vi "Protection_Valid_Calculation.vi"(8 "error in":errorcluster, 10 "Signal Settings":T1 {"Protection Configuration"."CRC Channels"."Data Type" items=["Signed", "Unsigned", "IEEE Float"]}, 11 "Signal Values In":dbl[](array[numeric])) -> (0 "error out":errorcluster, 3 "Signal Values Out":dbl[](array[numeric]))   [LabVIEW 2015, in "Protection and Counter Addon Engine.lvlib"]
uses:
  Protection and Counter Addon Engine.lvlib
  SubModules/Frame Protection Support/Source/Shared/Types/RT Exported Signal Settings.ctl
  SubModules/Frame Protection Support/Source/Shared/Types/Exported Counter Settings.ctl
  SubModules/Frame Protection Support/Source/Engine/Types/RT Protection Configuration.ctl
  SubModules/Frame Protection Support/Source/Shared/Types/Protection Type.ctl
  SubModules/Frame Protection Support/Source/Shared/Types/XNET Signal Configuration.ctl
  <vilib>/xnet/xnet.llb/XNET Convert (Signal to Frame Raw).vi
  SubModules/Frame Protection Support/Source/Shared/Protection and Counter Support Shared.lvlib
  SubModules/Frame Protection Support/Source/Engine/Protection and Counter Support Engine.lvlib
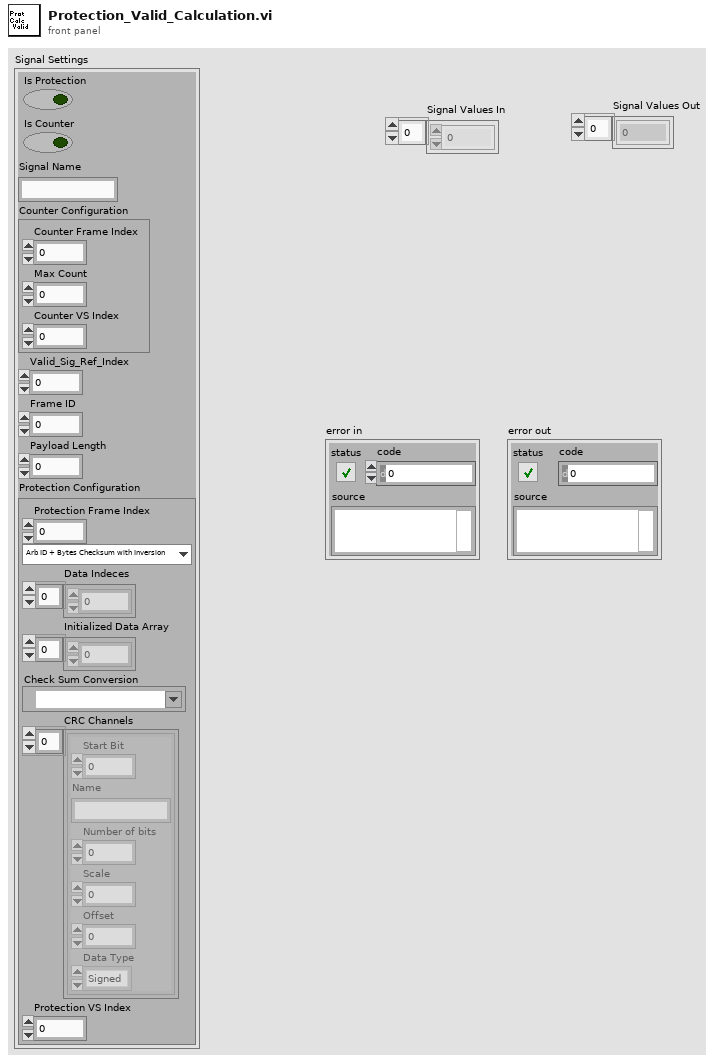
[diagram p1: front panel]
types:
  T1 = typedef "Protection and Counter Support Shared.lvlib/RT Exported Signal Settings.ctl" = cluster{"Is Protection":bool, "Is Counter":bool, "Signal Name":string, "Counter Configuration":T2, "Valid_Sig_Ref_Index":i32, "Frame ID":u32, "Payload Length":u32, "Protection Configuration":T3}
  T2 = typedef "Protection and Counter Support Shared.lvlib/Exported Counter Settings.ctl" = cluster{"Counter Frame Index":i32, "Max Count":dbl, "Counter VS Index":i32}
  T3 = typedef "Protection and Counter Support Engine.lvlib/RT Protection Configuration.ctl" = cluster{"Protection Frame Index":i32, "Protection Type":T4, "Data Indeces":i32[], "Initialized Data Array":dbl[], "Check Sum Conversion":refnum<k21>, "CRC Channels":T5[], "Protection VS Index":i32}
  T4 = typedef "Protection and Counter Support Shared.lvlib/Protection Type.ctl" = enum16{"Arb ID + Bytes Checksum with Inversion", "Arb ID + Bytes CRC with Inversion", "Reversed Raw Signal Checksum with Inversion"}
  T5 = typedef "Protection and Counter Support Shared.lvlib/XNET Signal Configuration.ctl" = cluster{"Start Bit":i32, "Name":string, "Number of bits":i32, "Scale":dbl, "Offset":dbl, "Data Type":u32}
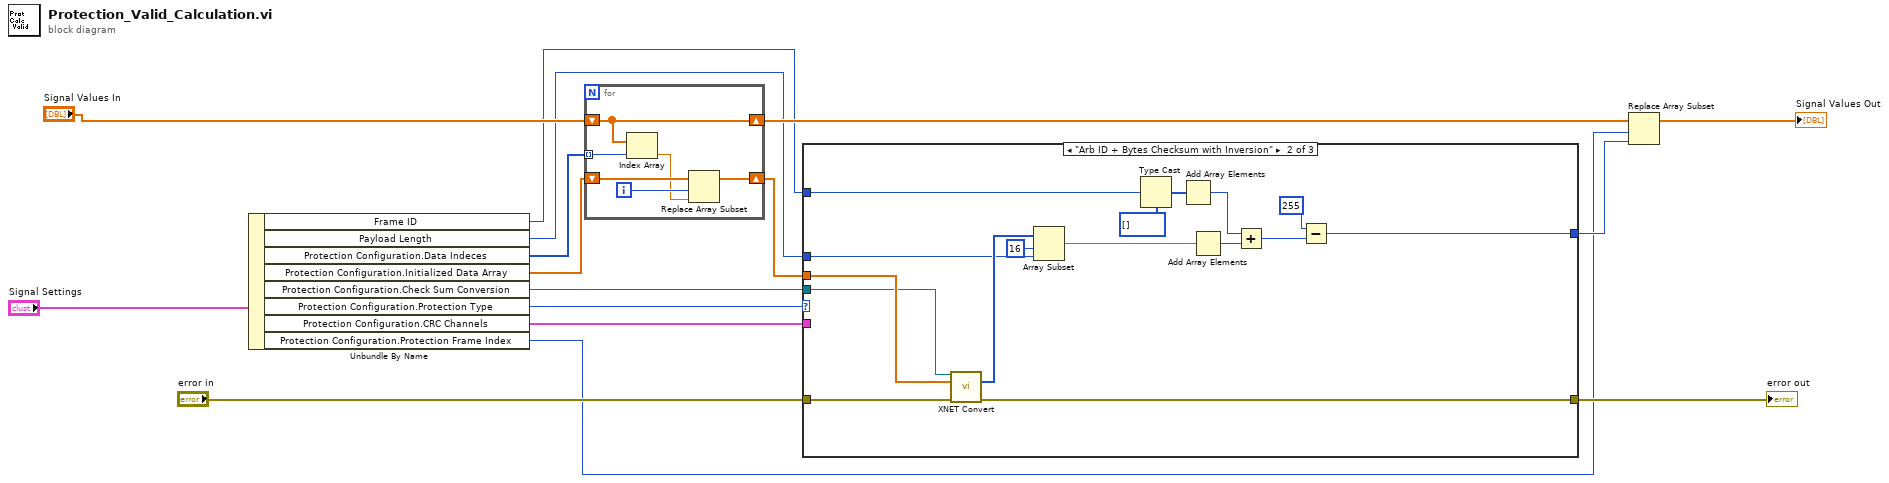
[diagram p0: block diagram]
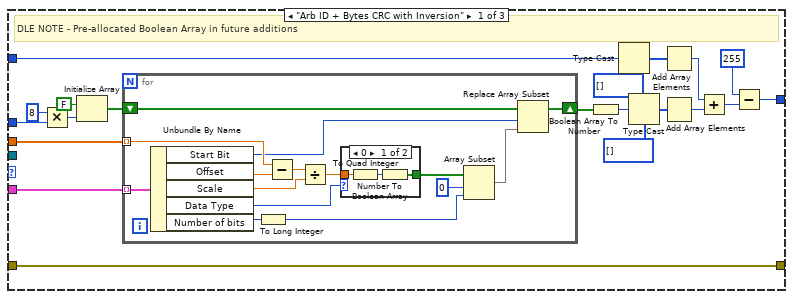
[diagram p2: hidden frame]
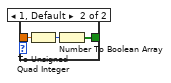
[diagram p3: hidden frame]
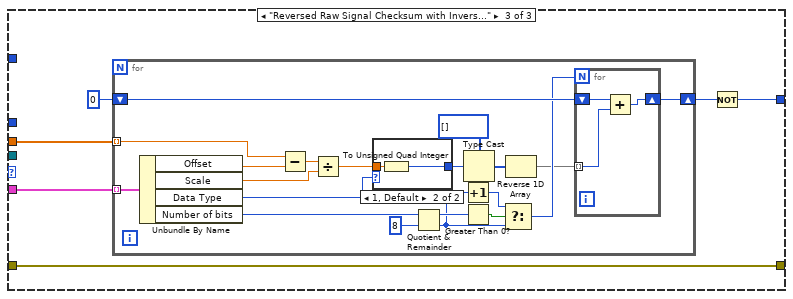
[diagram p4: hidden frame]
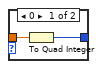
[diagram p5: hidden frame]
diagram:
  n1 = Unbundle By Name("Signal Settings") -> ("Frame ID"=w3:u32, "Payload Length"=w2:u32, "Protection Configuration.Data Indeces"=w11:i32[], "Protection Configuration.Initialized Data Array"=w9:dbl[], "Protection Configuration.Check Sum Conversion"=w5:refnum<k21>, "Protection Configuration.Protection Type"=w6:T4, "Protection Configuration.CRC Channels"=w12:T5[], "Protection Configuration.Protection Frame Index"=w4:i32)
  n2 = for {
    shift-right: [w21] -> w10
    shift-left: "Signal Values In" -> [w21]
    tunnel: w11 -> [w22] mode=indexing
    shift-right: [w17] -> w8
    shift-left: w9 -> [w20]
    i -> [w19]
    n3 = Index Array(array=w21, index=w22) -> (element=w18:dbl)
    n4 = Replace Array Subset(array=w20, new element=w18, index=w19) -> (w17:dbl[])
  }
  n5 = case shown="\"Arb ID + Bytes Checksum with Inversion\"" w6 {
    tunnel: w3 -> [w40 w77 _]
    tunnel: [w35 w72 w81] -> w7
    tunnel: "error in" -> [w31 w71 w80]
    tunnel: [w31 w70 w80] -> w15
    tunnel: w12 -> [w29 _ w83]
    tunnel: w8 -> [w30 w67 w82]
    tunnel: w5 -> [_ w66 _]
    tunnel: w2 -> [w25 w65 _]
    frame "Arb ID + Bytes CRC with Inversion" {
      # "DLE NOTE - Pre-allocated Boolean Array in future additions"
      n6 = Multiply(x=u32 8, y=w25) -> (x*y=w26:u32)
      n7 = Initialize Array(FALSE, w26) -> (w28:bool[])
      n8 = for {
        tunnel: w29 -> [w57] mode=indexing
        shift-right: [w48] -> w34
        shift-left: w28 -> [w50]
        tunnel: w30 -> [w47] mode=indexing
        n9 = Unbundle By Name(w57) -> ("Start Bit"=w44:i32, "Offset"=w56:dbl, "Scale"=w54:dbl, "Data Type"=w46:u32, "Number of bits"=w52:i32)
        n10 = To Long Integer(number=w52) -> (32bit integer=w43:i32)
        n11 = Subtract(x=w47, y=w56) -> (x-y=w55:dbl)
        n12 = Divide(x=w55, y=w54) -> (x/y=w53:dbl)
        n13 = case shown="0" w46 {
          tunnel: w53 -> [w60 w63]
          tunnel: [w58 w61] -> w45
          frame 0 {
            n14 = To Quad Integer(1:w60) -> (0:w59:i64)
            n15 = Number To Boolean Array(number=w59) -> (Boolean array=w58:bool[])
          }
          frame 1, Default {
            n16 = To Unsigned Quad Integer(1:w63) -> (0:w62:u64)
            n17 = Number To Boolean Array(number=w62) -> (Boolean array=w61:bool[])
          }
        }
        n18 = Array Subset(array=w45, index=0, length=w43) -> (w49:bool[])
        n19 = Replace Array Subset(array=w50, new element=w49, index=w44) -> (w48:bool[])
      }
      n20 = Boolean Array To Number(Boolean array=w34) -> (number=w33:u64)
      n21 = Type Cast(type=u8[] [], x=w40) -> (*(type *) &x=w39:u8[])
      n22 = Type Cast(type=u8[] [], x=w33) -> (*(type *) &x=w23:u8[])
      n23 = Add Array Elements(numeric array=w39) -> (sum=w38:u8)
      n24 = Add Array Elements(numeric array=w23) -> (sum=w42:u8)
      n25 = Add(x=w38, y=w42) -> (x+y=w37:u8)
      n26 = Subtract(x=u8 255, y=w37) -> (x-y=w35:u8)
    }
    frame "Arb ID + Bytes Checksum with Inversion" {
      n27 = call-poly <vilib>:"XNET Convert.vi"("session in"=w66, "signal data"=w67, "error in (no error)"=w71) -> ("frame data"=w68:u8[], "error out"=w70:errorcluster)  [unwired: 10 in, 1 out]
      n28 = Array Subset(array=w68, index=16 ("length"), length=w65) -> (w64:u8[])
      n29 = Type Cast(type=u8[] [], x=w77) -> (*(type *) &x=w76:u8[])
      n30 = Add Array Elements(numeric array=w76) -> (sum=w75:u8)
      n31 = Add Array Elements(numeric array=w64) -> (sum=w79:u8)
      n32 = Add(x=w75, y=w79) -> (x+y=w74:u8)
      n33 = Subtract(x=u8 255, y=w74) -> (x-y=w72:u8)
    }
    frame "Reversed Raw Signal Checksum with Inversion" {
      n34 = for {
        tunnel: w83 -> [w105] mode=indexing
        tunnel: w82 -> [w102] mode=indexing
        shift-right: [w99] -> w84
        shift-left: u8 0 -> [w100]
        n35 = Unbundle By Name(w105) -> ("Offset"=w104:dbl, "Scale"=w103:dbl, "Data Type"=w101:u32, "Number of bits"=w97:i32)
        n36 = Subtract(x=w102, y=w104) -> (x-y=w96:dbl)
        n37 = Divide(x=w96, y=w103) -> (x/y=w95:dbl)
        n38 = case shown="1, Default" w101 {
          tunnel: w95 -> [w110 w112]
          tunnel: [w109 w111] -> w98
          frame 0 {
            n39 = To Quad Integer(1:w110) -> (0:w109:i64)
          }
          frame 1, Default {
            n40 = To Unsigned Quad Integer(1:w112) -> (0:w111:u64)
          }
        }
        n41 = Quotient & Remainder(x=w97, y=8) -> (x-y*floor(x/y)=w92:i32, floor(x/y)=w90:i32)
        n42 = Increment(x=w90) -> (x+1=w91:i32)
        n43 = Greater Than 0?(x=w92) -> (x > 0?=w93:bool)
        n44 = Type Cast(type=u8[] [], x=w98) -> (*(type *) &x=w87:u8[])
        n45 = Select(t=w91, s=w93, f=w90) -> (s? t:f=w89:i32)
        n46 = Reverse 1D Array(array=w87) -> (reversed array=w86:u8[])
        n47 = for {
          N: w89 -> [_]
          tunnel: w86 -> [w107] mode=indexing
          shift-right: [w106] -> w99
          shift-left: w100 -> [w108]
          n48 = Add(x=w108, y=w107) -> (x+y=w106:u8)
        }
      }
      n49 = Not(x=w84) -> (.not. x?=w81:u8)
    }
  }
  "error out" <- w15
  n50 = Replace Array Subset(array=w10, new element=w7, index=w4) -> (→"Signal Values Out":dbl[])
